vi "Review Intermediate Result.vi"(0 "Vector 18GHz Path in":refnum<class "Vector 18GHz Path.lvclass">, 5 "One-Port Charact Data In":T1, 11 "error in (no error)":errorcluster) -> (4 "Vector 18GHz Path out":refnum<class "Vector 18GHz Path.lvclass">, 6 "Response":string, 8 "One-Port Charact Data Out":T1, 15 "error out":errorcluster)   [LabVIEW 2023, in "RFFixtureCharact.RFPM.lvlib" / "Vector 18GHz Path.lvclass"]
uses:
  Vector 18GHz Path.lvclass
  Vector 18GHz Path.lvclass/Vector 18GHz Path.ctl
  Public/Base Classes/Vector/Vector Abstract Path/Vector Abstract Path.lvclass
  Common/RFCalAndFixtureCharact.Common.lvlib
  Instruments/Cal Standard/Type Definitions/Standard Type.ctl
  Instruments/RFFixtureCharact.Instruments.lvlib
  Instruments/Cal Standard/Type Definitions/One-Port Charact Data.ctl
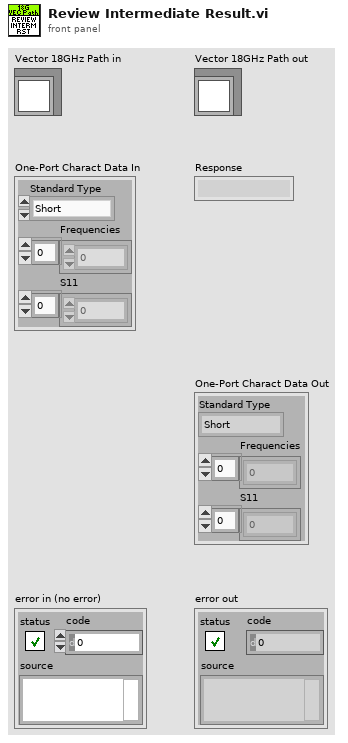
[diagram p1: front panel]
types:
  T1 = typedef "RFFixtureCharact.Instruments.lvlib/One-Port Charact Data.ctl" = cluster{"Standard Type":T2, "Frequencies":dbl[], "S11":cdb[]}
  T2 = typedef "RFFixtureCharact.Instruments.lvlib/Standard Type.ctl" = enum16{"Short", "Open", "Load", "PowerMeter", "None"}
  T3 = typedef "RFFixtureCharact.RFPM.lvlib/Vector 18GHz Path Group.lvclass/Sweep.ctl" = cluster{"Port Power":dbl, "Frequencies":dbl[], "Reference Level":dbl, "IF Bandwidth":dbl}
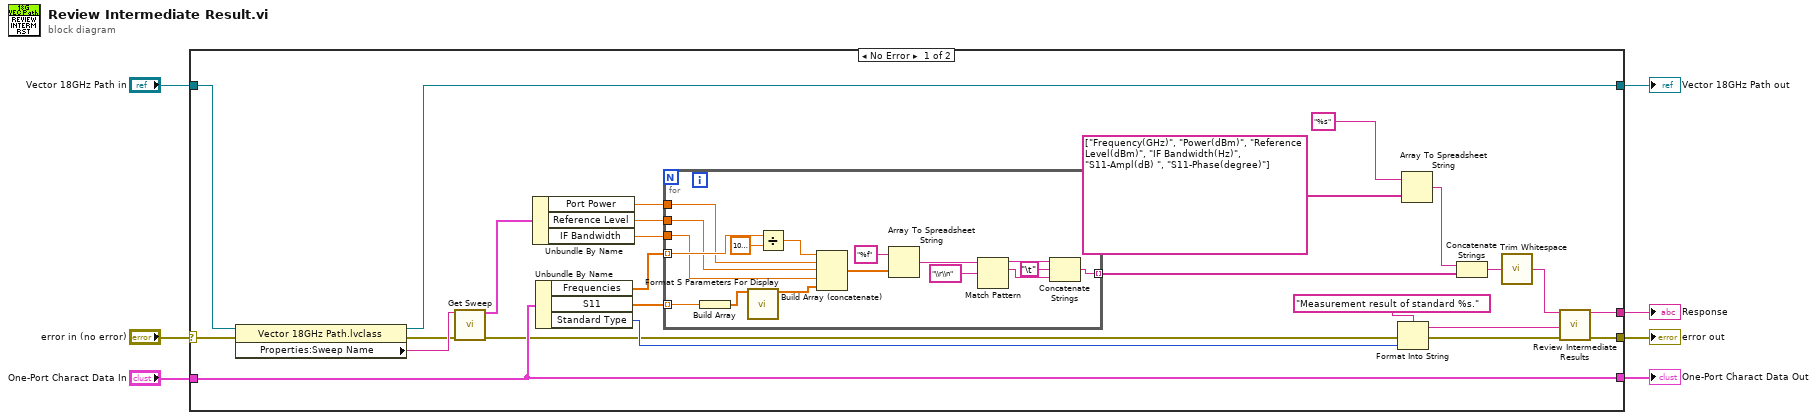
[diagram p0: block diagram]
diagram:
  n1 = case shown="No Error" "error in (no error)" {
    selector: "error in (no error)" -> [w14 w51]
    tunnel: [w23 w51] -> w5
    tunnel: [w24 _] -> w3
    tunnel: [w10 _] -> w4
    tunnel: "Vector 18GHz Path in" -> [w18 w50]
    tunnel: [w11 w50] -> w2
    tunnel: "One-Port Charact Data In" -> [w10 _]
    frame No Error {
      n2 = property class="Vector 18GHz Path.lvclass"(reference=w18, error in=w14) -> (reference out=w11:refnum<class "Vector 18GHz Path.lvclass">, error out=w15:errorcluster, "Properties:Sweep Name"=w16:string)
      n3 = call "Get Sweep.vi"("Sweep Name"=w16, "error in (no error)"=w15) -> ("Grid"=w17:T3, "error out"=w9:errorcluster)  [unwired: 11 in, 1 out]
      n4 = Unbundle By Name(w17) -> ("Port Power"=w8:dbl, "Reference Level"=w13:dbl, "IF Bandwidth"=w12:dbl)
      n5 = Unbundle By Name(w10) -> ("Frequencies"=w26:dbl[], "S11"=w27:cdb[], "Standard Type"=w20:T2)
      n6 = for {
        tunnel: [w40] -> w29 mode=indexing
        tunnel: w27 -> [w38] mode=indexing
        tunnel: w26 -> [w36] mode=indexing
        tunnel: w8 -> [w35]
        tunnel: w12 -> [w33]
        tunnel: w13 -> [w34]
        n7 = Build Array(w38) -> (w37:cdb[])
        n8 = call "Format S Parameters For Display.vi"("S Parameters"=w37) -> ("S Parameters For Display"=w39:dbl[])  [unwired: 14 in]
        n9 = Divide(x=w36, y=1000000000.0) -> (x/y=w48:dbl)
        n10 = Build Array (concatenate)(w48, w35, w34, w33, w39) -> (w44:dbl[])
        n11 = Array To Spreadsheet String(array=w44, 3:"%f" ("format string")) -> (spreadsheet string=w46:string)  [unwired: 1 in]
        n12 = Match Pattern(string=w46, regular expression="\\r\\n") -> (before substring=w43:string, match substring=w41:string)  [unwired: 1 in, 2 out]
        n13 = Concatenate Strings(w43, "\t", w41) -> (w40:string)
      }
      n14 = Format Into String(format string="Measurement result of standard %s." ("Request Header"), error in=w9, w20) -> (resulting string=w19:string, error out=w22:errorcluster)  [unwired: 1 in]
      n15 = Array To Spreadsheet String(array=string[] ["Frequency(GHz)", "Power(dBm)", "Reference Level(dBm)", "IF Bandwidth(Hz)", "S11-Ampl(dB) ", "S11-Phase(degree)"], 3:"%s" ("format string")) -> (spreadsheet string=w30:string)  [unwired: 1 in]
      n16 = Concatenate Strings(w30, w29) -> (w28:string)
      n17 = call <vilib>:"Trim Whitespace.vi"("string"=w28) -> ("trimmed string"=w25:string)  [unwired: 1 in]
      n18 = call "Review Intermediate Results.vi"("Intermediate Results"=w25, "Request Header"=w19, "error in (no error)"=w22) -> ("Response"=w24:string, "error out"=w23:errorcluster)  [unwired: 11 in]
    }
    frame Error {
    }
  }
  "error out" <- w5
  "Vector 18GHz Path out" <- w2
  "Response" <- w3
  "One-Port Charact Data Out" <- w4
